vi "702_1_f_cor.vi"() -> ()   [LabVIEW 2010]
panel:
  out "f":dbl
  in  "b":dbl
  in  "x":dbl
  in  "a":dbl
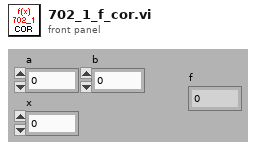
[diagram p1: front panel]
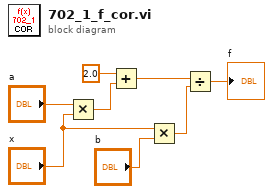
[diagram p0: block diagram]
diagram:
  n1 = Multiply(x="a", y="x") -> (x*y=w7:dbl)
  n2 = Add(x=2.0, y=w7) -> (x+y=w6:dbl)
  n3 = Multiply(x="x", y="b") -> (x*y=w2:dbl)
  n4 = Divide(x=w6, y=w2) -> (x/y=→"f":dbl)
